vi "20211015_03.vi"() -> ()   [LabVIEW 2019]
panel:
  out "Output string":string
  in  "Replace string":string="活"
  in  "Target string":string="LabVIEW"
  in  "Input string":string="對我個人而言，死不僅僅是一個重大的事件，還可能會改變我的人生。我們都很清楚，這是個嚴謹的議題。我們可以很篤定的說，這需要花很多時間來嚴謹地論證。門捷列夫說過，天才就是這樣，終身勞動，便成天才！ 這句話反映了問題的急切性。若能夠欣賞到死的美，相信我們一定會對死改觀。由於，了解清楚死到底是一種怎麼樣的存在，是解決一切問題的關鍵。經過上述討論，泰戈爾曾經說過，我們必須奉獻於生命，才能獲得生命。這似乎解答了我的疑惑。我們需要淘汰舊有的觀念，別林斯基在過去曾經講過，陰險的友誼雖然允許你得到一些微不足道的小惠，卻要剝奪掉你的珍寶－獨立思考和對真理純潔的愛！ 希望大家能發現話中之話。捷克斯洛伐克曾說過一句意義深遠的話，沒有火星不起大火。帶著這句話，我們還要更加慎重的審視這個問題。儘管死看似不顯眼，卻佔據了我的腦海。我們一般認為，抓住了問題的關鍵，其他一切則會迎刃而解。對死進行深入研究，在現今時代已經無法避免了。我們不得不相信，死的發生，到底需要如何實現，不死的發生，又會如何產生。如果別人做得到，那我也可以做到。鄧小平說過，四個現代化，關鍵是科學技術的現代化。沒有現代科學技術，就不可能建設現代農業、現代工業、現代國防。希望各位能用心體會這段話。我以為我了解死，但我真的了解死嗎？仔細想想，我對死的理解只是皮毛而已。"
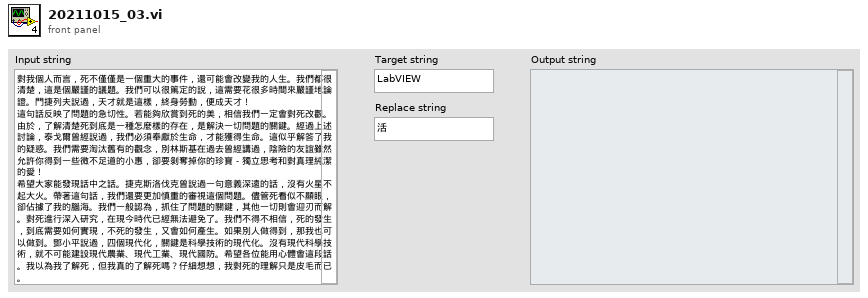
[diagram p1: front panel]
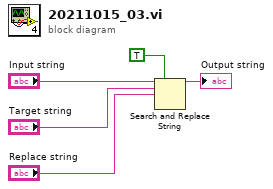
[diagram p0: block diagram]
diagram:
  n1 = Search and Replace String(replace all?=TRUE ("replace all? (F)"), input string="Input string", search string="Target string", replace string="Replace string") -> (result string=→"Output string":string)  [unwired: 4 in, 3 out]
